vi "Notify Set Previous Button Visibility.vi"(8 "error in (no error)":errorcluster, 10 "Event Data":bool, 11 "Project View in":refnum<class "Project View.lvclass">) -> (0 "error out":errorcluster, 3 "Project View out":refnum<class "Project View.lvclass">)   [LabVIEW 2013, in "Project View.lvlib" / "Project View.lvclass"]
uses:
  Project View.lvclass
  Project View.lvclass/Project View.ctl
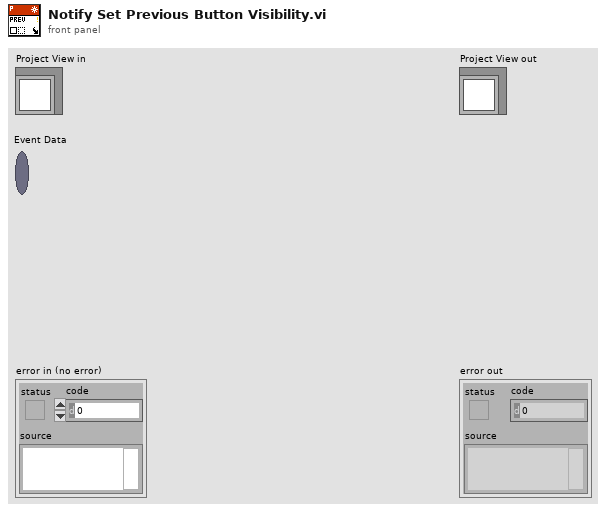
[diagram p1: front panel]
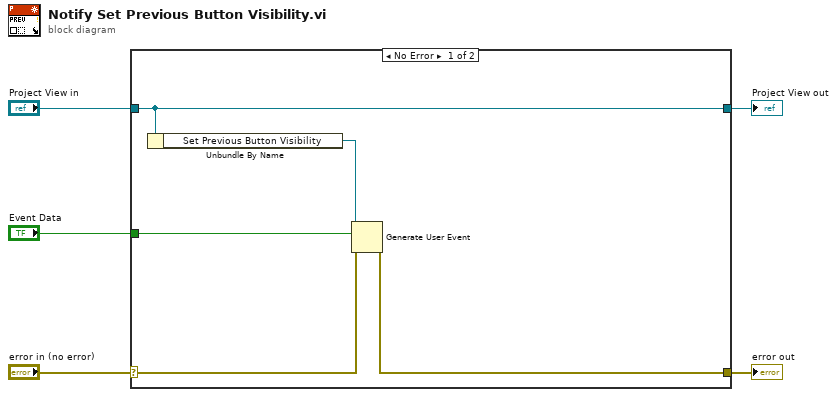
[diagram p0: block diagram]
diagram:
  n1 = case shown="No Error" "error in (no error)" {
    selector: "error in (no error)" -> [w7 w12]
    tunnel: [w6 w12] -> w4
    tunnel: [w10 w11] -> w2
    tunnel: "Project View in" -> [w10 w11]
    tunnel: "Event Data" -> [w8 _]
    frame No Error {
      n2 = Unbundle By Name(w10) -> ("Set Previous Button Visibility"=w9:refnum<user-event>)
      n3 = Generate User Event(user event=w9, event data cluster=w8, error in=w7) -> (error out=w6:errorcluster)  [unwired: 1 in, 1 out]
    }
    frame Error {
    }
  }
  "error out" <- w4
  "Project View out" <- w2
